vi "Monitor.vi"() -> ()   [LabVIEW 2020]
uses:
  Types/States.ctl
  NotifyIcon/TypeDefs/NotifyIcon Events.ctl
  NotifyIcon/TypeDefs/NotifyIcon Event Registration Actions.ctl
  <vilib>/nisyscfg/Close (System).vi
  <vilib>/addons/database/Connection.llb/DB Tools Open Connec (Path).vi
  <vilib>/regexp/Match Regular Expression.xnode
  <vilib>/nisyscfg/nisyscfg.lvlib
  <resource>/objmgr/nisysapi.rc
  <resource>/objmgr/nicontrollersysapi.rc
  <vilib>/addons/database/NI_Database_API.lvlib
panel:
  out "Icon Path":path
  in  "stop":bool
  out "Last error":errorcluster
  out "IP Address":string
  out "HostName":string
  out "Local Device List":string[][](table)
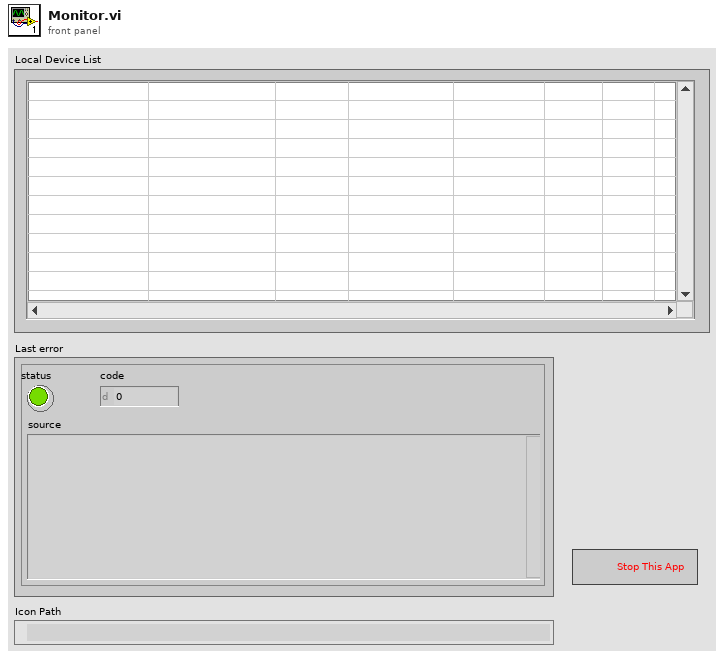
[diagram p1: front panel]
types:
  T1 = enum32{"Invalid", "Standard", "Closed", "Hidden", "Minimized", "Maximized"}
  T2 = typedef "NotifyIcon Event Registration Actions.ctl" = enum16{"Initial Event Registration", "Add to Event Registration", "Destroy Events and Re-register"}
  T3 = typedef "NotifyIcon Events.ctl" = enum16{"BalloonTipClicked", "BalloonTipClosed", "BalloonTipShown", "Click", "Disposed", "DoubleClick", "MouseClick", "MouseDoubleClick", "MouseDown", "MouseMove", "MouseUp", "MenuItemClick", "MenuItemSelect"}
  T4 = typedef "States.ctl" = enum16{"List Devices", "Log DB", "Wait"}
  T5 = typedef "NI_Database_API.lvlib/Conn ObjectReference.ctl" = refnum<k1>
  T6 = typedef "NotifyIcon Event Data.ctl" = cluster{"NotifyIcon Event":T3, "Data String":string}
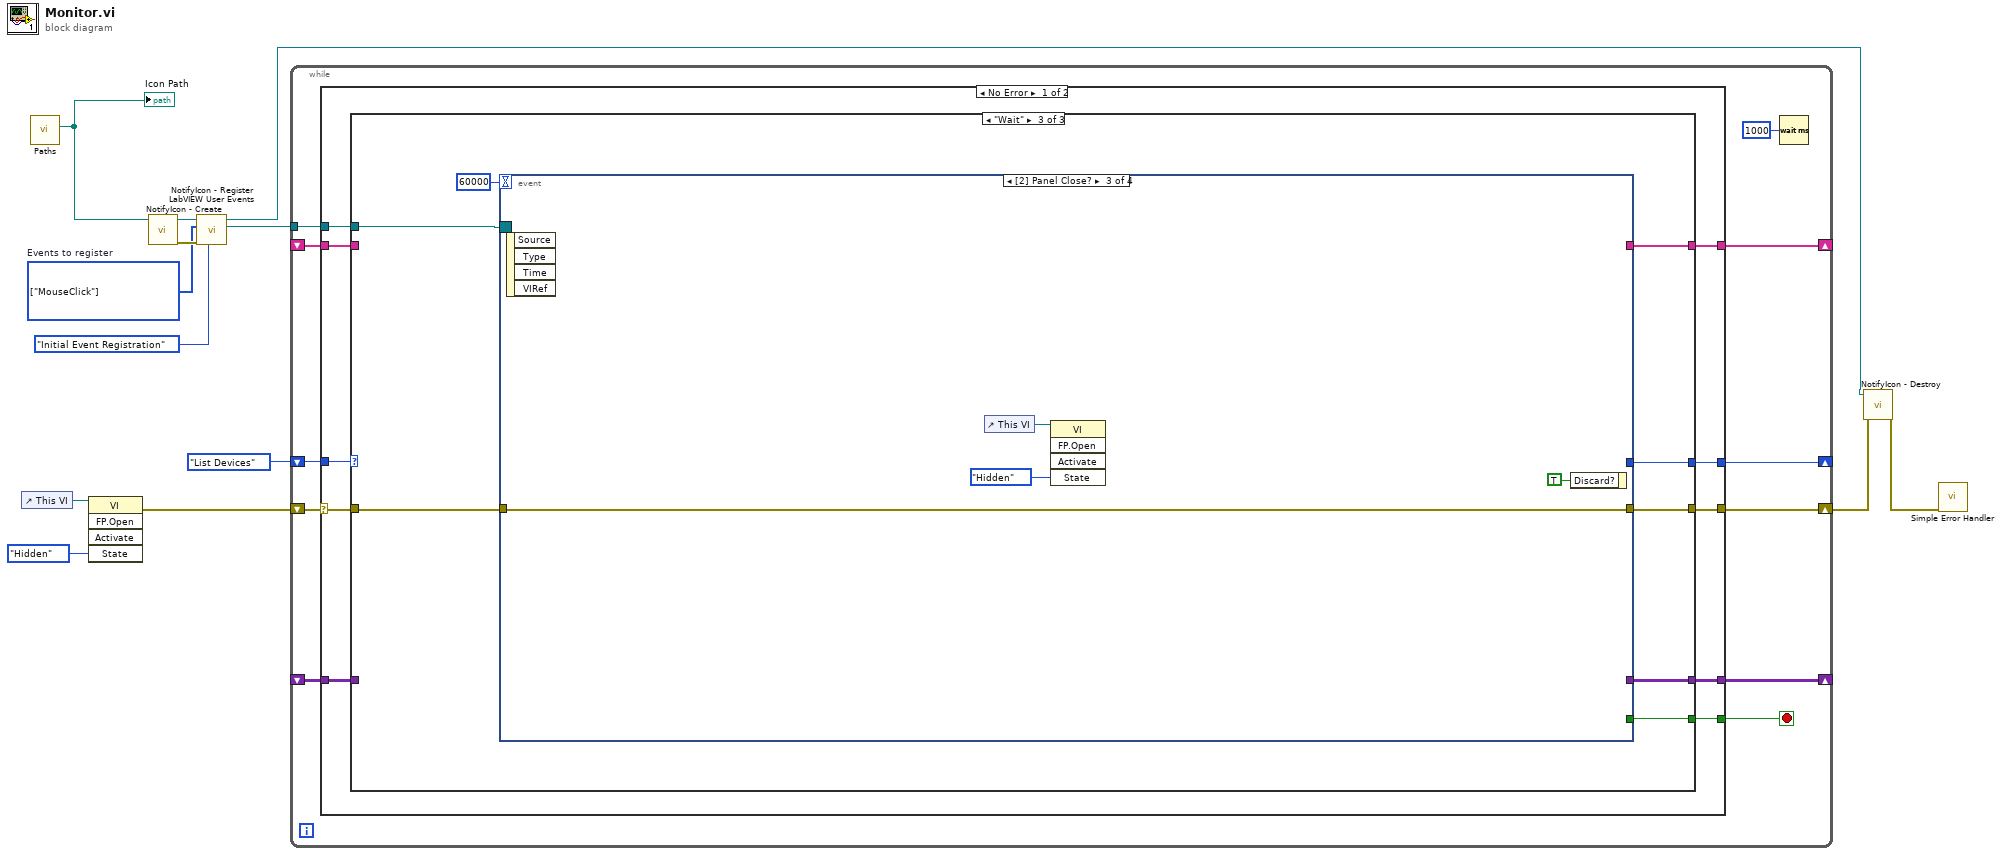
[diagram p0: block diagram]
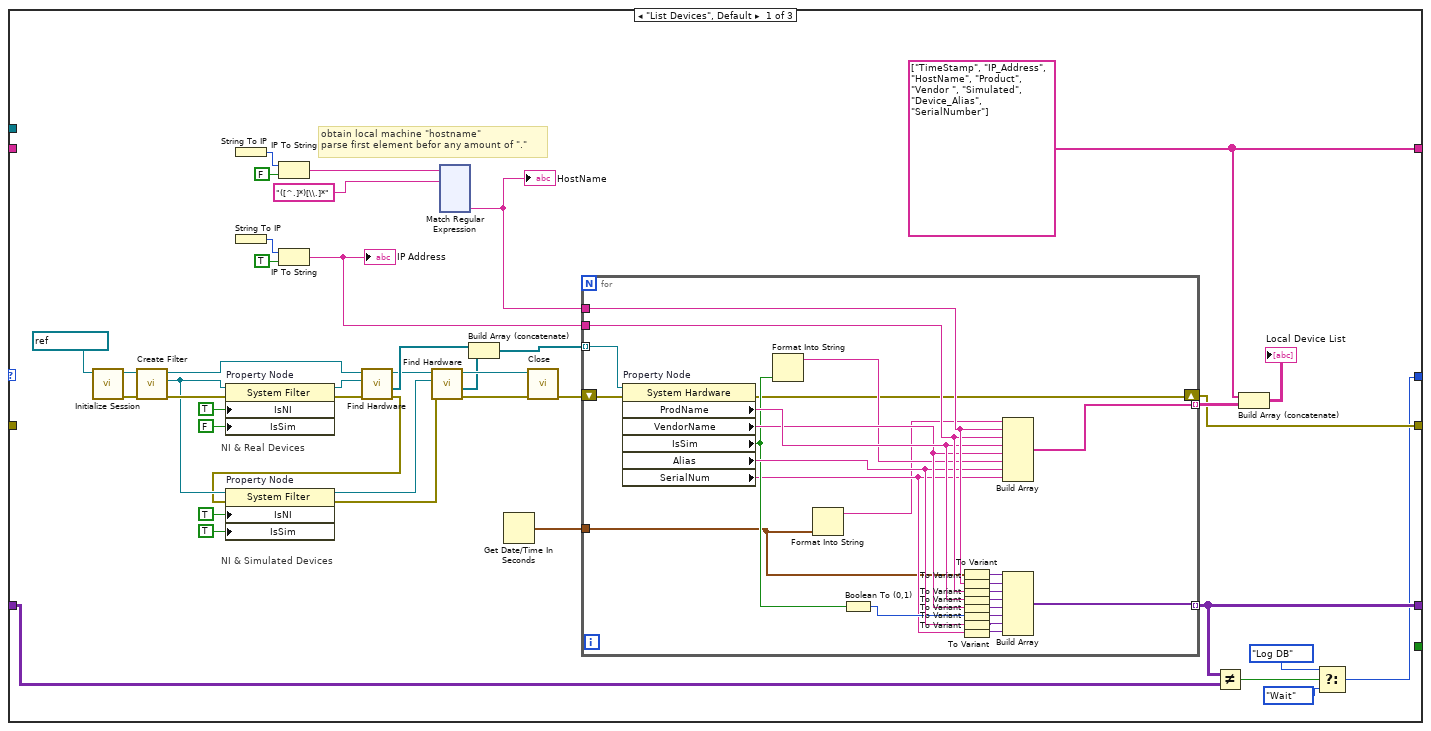
[diagram p2: hidden frame]
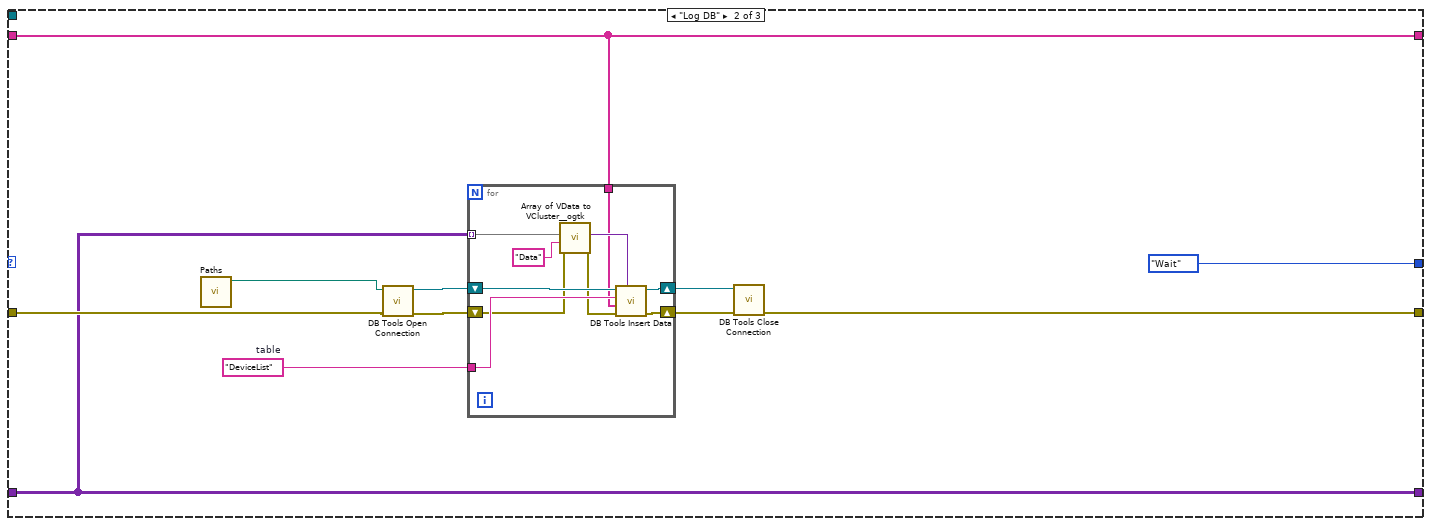
[diagram p3: hidden frame]
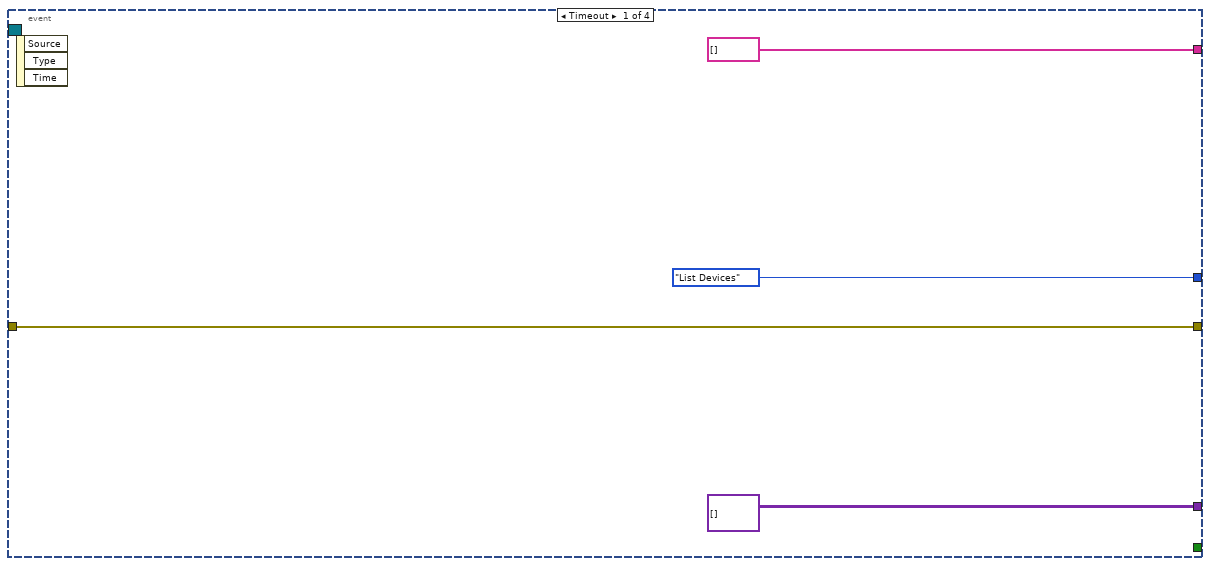
[diagram p4: hidden frame]
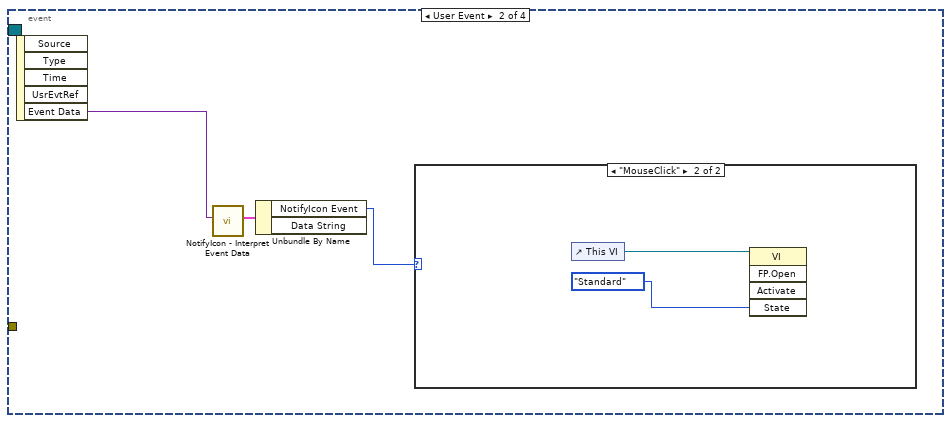
[diagram p5: hidden frame]
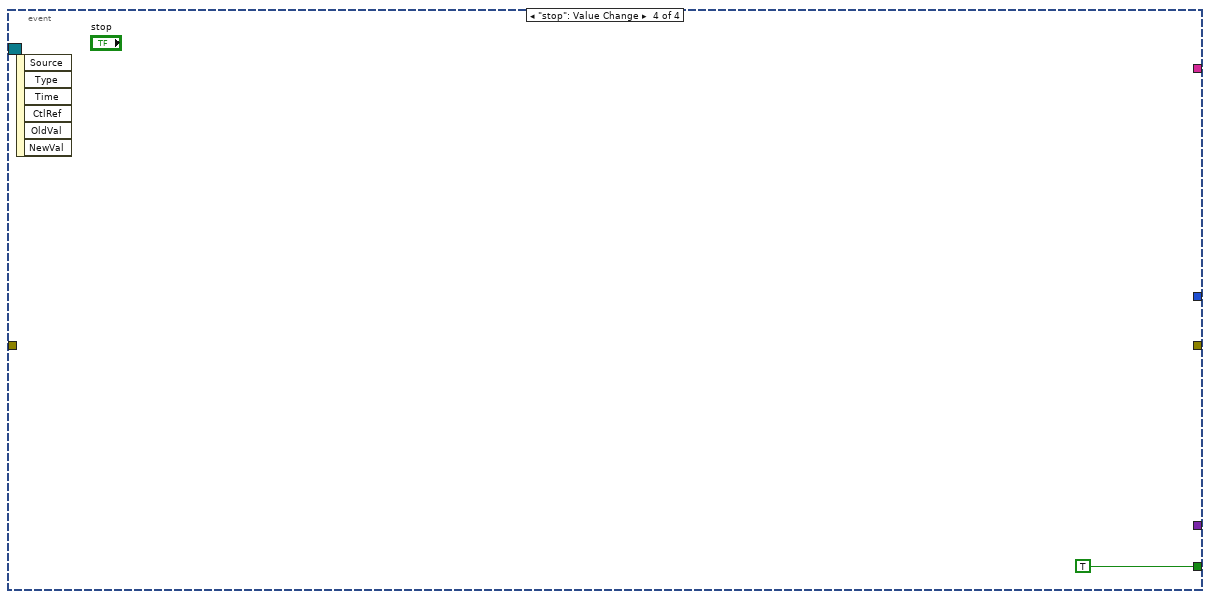
[diagram p7: hidden frame]
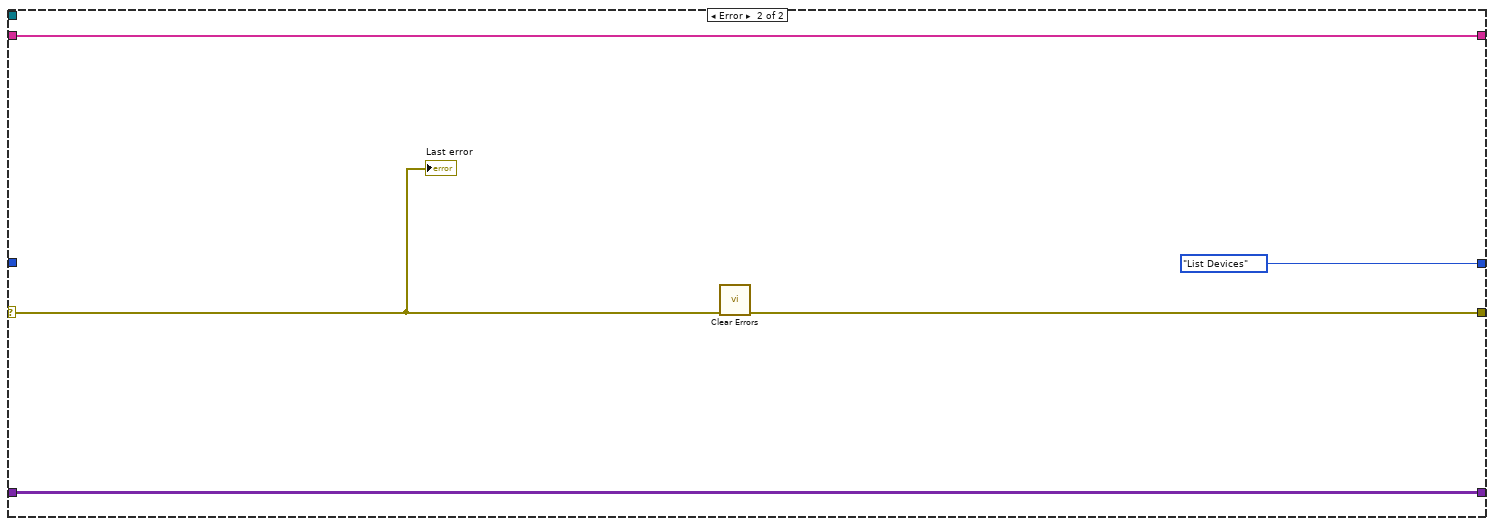
[diagram p8: hidden frame]
diagram:
  w8 = T3[] [enum."MouseClick"] items=["BalloonTipClicked", "BalloonTipClosed", "BalloonTipShown", "Click", "Disposed", "DoubleClick", "MouseClick", "MouseDoubleClick", "MouseDown", "MouseMove", "MouseUp", "MenuItemClick", "MenuItemSelect"]  # Events to register
  n1 = control-ref of="This VI"() -> (w2:refnum<vi>)
  n2 = call "Paths.vi"() -> ("Icon Path"=w7:path)  [unwired: 10 in, 1 out]
  "Icon Path" <- w7
  n3 = invoke class="VI" method="FP.Open"(reference=w2, "State"=T1."Hidden") -> (error out=w1:errorcluster)  [unwired: 3 in, 4 out]
  n4 = call "NotifyIcon - Create.vi"("Icon File Path"=w7) -> ("error out"=w12:errorcluster, "NotifyIcon reference"=w11:refnum<k24>)  [unwired: 9 in]
  n5 = call "NotifyIcon - Register LabVIEW User Events.vi"("Action"=NotifyIcon_Event_Registration_Actions."Initial Event Registration", "error in"=w12, "Events to register"=w8, "NotifyIcon reference in"=w11) -> ("Event Registration Refnum"=w9:refnum<event-registration>, "NotifyIcon reference out"=w4:refnum<k24>)  [unwired: 5 in, 1 out]
  n6 = while {
    shift-right: [w23] -> _
    shift-left: _ -> [w22]
    shift-right: [w17] -> w6
    shift-left: w1 -> [w21]
    shift-right: [w20] -> _
    shift-left: _ -> [w19]
    shift-right: [w18] -> _
    shift-left: States."List Devices" -> [w24]
    tunnel: w9 -> [w15]
    stop <- w14 stop-if-true
    n7 = case shown="No Error" w21 {
      selector: w21 -> [w31 w261]
      tunnel: w24 -> [w34 _]
      tunnel: [w33 w260] -> w23
      tunnel: w22 -> [w32 w260]
      tunnel: [w30 w259] -> w20
      tunnel: w19 -> [w29 w259]
      tunnel: [w28 States."List Devices"] -> w18
      tunnel: [w27 w263] -> w17
      tunnel: w15 -> [w26 _]
      tunnel: [w25 _] -> w14
      frame No Error {
        n8 = case shown="\"Wait\"" w34 {
          tunnel: [w50 w216 w243] -> w33
          tunnel: [w54 w221 w240] -> w27
          tunnel: w32 -> [w51 w216 _]
          tunnel: w31 -> [_ w219 w241]
          tunnel: [w52 w218 w242] -> w30
          tunnel: w29 -> [_ w218 _]
          tunnel: [w46 States."Wait" w244] -> w28
          tunnel: w26 -> [_ _ w238]
          tunnel: [_ _ w237] -> w25
          frame "List Devices", Default {
            w52 = string[] ["TimeStamp", "IP_Address", "HostName", "Product", "Vendor ", "Simulated", "Device_Alias", "SerialNumber"] ("array")
            # "NI & Real Devices"
            # "NI & Simulated Devices"
            # "obtain local machine \"hostname\" \nparse first element befor any amount of \".\""
            n9 = call <vilib>:"Initialize Session.vi"("Target (localhost)"=refnum<k21> "localhost") -> ("error out"=w73:errorcluster, "Session out"=w74:refnum<k21>)  [unwired: 9 in]
            n10 = call <vilib>:"Create Filter.vi"("error in (no error)"=w73, "Session in"=w74) -> ("error out"=w75:errorcluster, "Filter out"=w38:refnum<k20>, "Session out"=w70:refnum<k21>)  [unwired: 7 in]
            n11 = property on="Property Node" class="System Filter"(reference=w38, error in=w75, "IsNI"=TRUE ("Devices & Chassis:Is NI Product"), "IsSim"=FALSE ("Devices & Chassis:Is Simulated")) -> (reference out=w71:refnum<k20>, error out=w72:errorcluster)
            n12 = String To IP() -> (0:w62:u32)  [unwired: 1 in]
            n13 = String To IP() -> (0:w58:u32)  [unwired: 1 in]
            n14 = IP To String(1:FALSE ("dot notation? (F)"), 2:w62) -> (0:w63:string)
            n15 = IP To String(1:TRUE ("dot notation? (F)"), 2:w58) -> (0:w57:string)
            "IP Address" <- w57
            n16 = call <vilib>:"Find Hardware.vi"("error in (no error)"=w72, "Filter in"=w71, "Session in"=w70) -> ("error out"=w36:errorcluster, "Resources out"=w68:refnum<k20>[], "Session out"=w45:refnum<k21>)  [unwired: 5 in, 1 out]
            n17 = property on="Property Node" class="System Filter"(reference=w38, error in=w36, "IsNI"=TRUE ("Devices & Chassis:Is NI Product"), "IsSim"=TRUE ("Devices & Chassis:Is Simulated")) -> (reference out=w37:refnum<k20>, error out=w35:errorcluster)
            n18 = call <vilib>:"Find Hardware.vi"("error in (no error)"=w35, "Filter in"=w37, "Session in"=w45) -> ("error out"=w44:errorcluster, "Resources out"=w41:refnum<k20>[], "Session out"=w43:refnum<k21>)  [unwired: 5 in, 1 out]
            n19 = xnode "Match Regular Expression"("input string"=w63, "regular expression"="([^.]*)[\\.]*") -> ("submatch 1"=w56:string)  [unwired: 4 in, 5 out]
            "HostName" <- w56
            n20 = Build Array (concatenate)(w68, w41) -> (w42:refnum<k20>[])
            n21 = Get Date/Time In Seconds() -> (seconds since 1Jan1904=w55:timestamp)
            n22 = call-poly <vilib>:"Close.vi"("error in (no error)"=w44, "Session in"=w43) -> ("error out"=w67:errorcluster)  [unwired: 9 in]
            n23 = for {
              tunnel: w42 -> [w214] mode=indexing
              tunnel: [w213] -> w66 mode=indexing
              tunnel: w57 -> [w204]
              tunnel: w56 -> [w205]
              tunnel: w55 -> [w194]
              tunnel: [w193] -> w50 mode=indexing
              shift-right: [w192] -> w54
              shift-left: w67 -> [w215]
              n24 = property on="Property Node" class="System Hardware"(reference=w214, error in=w215) -> (error out=w192:errorcluster, "ProdName"=w203:string, "VendorName"=w202:string, "IsSim"=w199:bool, "Alias"=w200:string, "SerialNum"=w196:string)  [unwired: 1 out]
              n25 = Format Into String "Format Into String"(w199) -> (resulting string=w201:string)  [unwired: 3 in, 1 out]
              n26 = Format Into String "Format Into String"(w194) -> (resulting string=w195:string)  [unwired: 3 in, 1 out]
              n27 = Boolean To (0,1)(Boolean=w199) -> (0, 1=w198:i16)
              n28 = To Variant(anything=w194) -> (Variant=w212:variant)
              n29 = To Variant(anything=w205) -> (Variant=w211:variant)
              n30 = To Variant(anything=w204) -> (Variant=w210:variant)
              n31 = To Variant(anything=w203) -> (Variant=w209:variant)
              n32 = To Variant(anything=w202) -> (Variant=w208:variant)
              n33 = To Variant(anything=w198) -> (Variant=w207:variant)
              n34 = To Variant(anything=w200) -> (Variant=w206:variant)
              n35 = To Variant(anything=w196) -> (Variant=w197:variant)
              n36 = Build Array "Build Array"(w195, w205, w204, w203, w202, w201, w200, w196) -> (w213:string[])
              n37 = Build Array "Build Array"(w212, w211, w210, w209, w208, w207, w206, w197) -> (w193:variant[])
            }
            n38 = Not Equal?(x=w50, y=w51) -> (x != y?=w49:bool)
            n39 = Build Array (concatenate)(w52, w66) -> (→"Local Device List":string[][])
            n40 = Select(t=States."Log DB", s=w49, f=States."Wait") -> (s? t:f=w46:T4)
          }
          frame "Log DB" {
            w222 = "DeviceList"  # table
            n41 = call "Paths.vi"() -> ("UDL Path"=w223:path)  [unwired: 10 in, 1 out]
            n42 = call-poly <vilib>:"DB Tools Open Connection.vi"("error in (no error)"=w219, "connection information"=w223) -> ("error out"=w220:errorcluster, "connection reference"=w224:T5)  [unwired: 6 in]
            n43 = for {
              tunnel: w222 -> [w232]
              tunnel: w216 -> [w231] mode=indexing
              shift-right: [w236] -> w226
              shift-left: w224 -> [w234]
              shift-right: [w235] -> w225
              shift-left: w220 -> [w229]
              tunnel: w218 -> [w227]
              n44 = call <userlib>:"Array of VData to VCluster__ogtk.vi"("error in (no error)"=w229, "Cluster Name"="Data", "Array"=w231) -> ("error out"=w228:errorcluster, "VCluster"=w230:variant)  [unwired: 7 in]
              n45 = call <vilib>:"DB Tools Insert Data.vi"("data"=w230, "error in (no error)"=w228, "columns"=w227, "table"=w232, "connection reference"=w234) -> ("error out"=w235:errorcluster, "connection reference out"=w236:T5)  [unwired: 5 in]
            }
            n46 = call <vilib>:"DB Tools Close Connection.vi"("error in (no error)"=w225, "connection reference"=w226) -> ("error out"=w221:errorcluster)  [unwired: 5 in]
          }
          frame "Wait" {
            n47 = event shown="[2] Panel Close?" {
              selector: w238 -> [_ _ _ _]
              dyn-events: _ -> [_ _ _ _]
              timeout: 60000 -> [_ _ _ _]
              tunnel: [States."List Devices" _ _ _] -> w244
              tunnel: [variant[][] [] _ _ _] -> w243
              tunnel: [string[] [] ("array") _ _ _] -> w242
              tunnel: w241 -> [w245 _ w256 _]
              tunnel: [w245 _ w256 _] -> w240
              tunnel: [_ _ _ TRUE] -> w237
              event Timeout {
                n48 = event-data() -> ()  [unwired: 1 in, 3 out]
              }
              event User Event {
                n49 = event-data() -> ("Event Data"=w250:variant)  [unwired: 1 in, 4 out]
                n50 = call "NotifyIcon - Interpret Event Data.vi"("NotifyIcon Event Data"=w250) -> ("NotifyIcon Event Data"=w251:T6)  [unwired: 9 in, 1 out]
                n51 = Unbundle By Name(w251) -> ("NotifyIcon Event"=w249:T3)  [unwired: 1 out]
                n52 = case shown="\"MouseClick\"" w249 {
                  frame "BalloonTipClicked", Default {
                  }
                  frame "MouseClick" {
                    n53 = control-ref of="This VI"() -> (w253:refnum<vi>)
                    n54 = invoke class="VI" method="FP.Open"(reference=w253, "State"=T1."Standard" ("Front Panel Window:State")) -> ()  [unwired: 3 in, 5 out]
                  }
                }
              }
              event Panel Close? {
                n55 = event-data() -> ()  [unwired: 1 in, 4 out]
                n56 = control-ref of="This VI"() -> (w255:refnum<vi>)
                n57 = invoke class="VI" method="FP.Open"(reference=w255, "State"=T1."Hidden") -> ()  [unwired: 3 in, 5 out]
                n58 = event-data("Discard?"=TRUE) -> ()  [unwired: 1 in, 1 out]
              }
              event "stop": Value Change {
                n59 = event-data() -> ()  [unwired: 1 in, 6 out]
              }
            }
          }
        }
      }
      frame Error {
        n60 = call <vilib>:"Clear Errors.vi"("error in (no error)"=w261) -> ("error out"=w263:errorcluster)  [unwired: 5 in, 1 out]
        "Last error" <- w261
      }
    }
    n61 = Wait (ms)(milliseconds to wait=u32 1000) -> ()  [unwired: 1 out]
  }
  n62 = call "NotifyIcon - Destroy.vi"("error in"=w6, "NotifyIcon reference"=w4) -> ("error out"=w5:errorcluster)  [unwired: 9 in]
  n63 = call <vilib>:"Simple Error Handler.vi"("error in (no error)"=w5) -> ()  [unwired: 4 in, 5 out]
